vi "Configure.vi"(8 "error in":errorcluster, 10 "name":string, 11 "nPAS in":refnum<class "nPAS.lvclass">) -> (0 "error out":errorcluster, 3 "nPAS out":refnum<class "nPAS.lvclass">)   [LabVIEW 2015, in "nPAS.lvclass"]
doc: "Configure the instrument class. If there is no config file specified, an error"
uses:
  nPAS.lvclass
  Session/Raw FPGA/FPGA Session.lvclass
  Session/Raw FPGA/FPGA Session.lvclass/FPGA Session.ctl
  Reusable/Instrument/Instrument.lvclass/Instrument.ctl
  Reusable/PAS/Main/PAS.lvclass/PAS.ctl
  nPAS.lvclass/nPAS.ctl
  Session/Raw FPGA/Read FPGA Ref.vi
  Reusable/Instrument/Read Cfg Session.vi
  Reusable/PAS/Main/Read Chirp.vi
  Reusable/Instrument/Read Log Session.vi
  Reusable/PAS/Main/Get Speaker State.vi
  <vilib>/Utility/config.llb/Read Key (Double).vi
  <vilib>/Utility/config.llb/Read Key (String).vi
  <vilib>/rvi/interface/common/niFpgaWaitOnOcc.vi
  <vilib>/Utility/error.llb/Error Cluster From Error Code.vi
  <vilib>/rvi/errors/niLvFpgaAdjustHostInterfaceError.vi
  Reusable/PAS/Main/PAS.lvclass
  FPGA Ref.ctl
  <userlib>/_Session Fwk/Session - Root.lvclass
  <vilib>/rvi/interface/nirviMethod/nirviMethod.xnode
  FPGA Bitfiles/NickIO.lvbitx
  <vilib>/rvi/interface/nirviReadWriteControl/nirviReadWriteControl.xnode
  FPGA/PAS Modulation.ctl
  <vilib>/FPGAPlugInAG/cRIO-9081/niLvFpga_ConfigureFifo_cRIO-9081.vi
  <vilib>/rvi/errors/niLvFpgaMergeErrorWithErrorCode.vi
  <vilib>/FPGAPlugInAG/cRIO-9081/niLvFpga_StartFifo_cRIO-9081.vi
  Reusable/Session Log/System Log.lvclass
  Reusable/Session APIs/File Access/Config Data/Config Data.lvclass
  <vilib>/Utility/config.llb/NI_LVConfig.lvlib
  NiFpgaLv.dll
  <vilib>/FPGAPlugInAG/cRIO-9081/niLvFpga_WriteFifo_cRIO-9081.vi
panel:
  out "Actual Depth 2":u32
  out "Actual Depth":u32
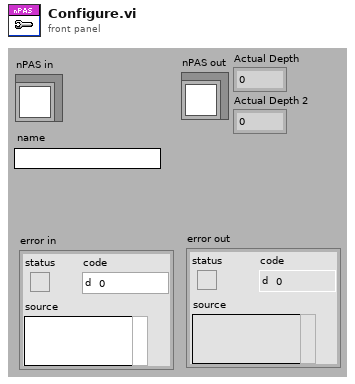
[diagram p1: front panel]
types:
  T1 = cluster{"f0":fxp<+,32,0>, "Mod":enum16{"Sine", "Square"}, "Vscale":fxp<+,32,0>, "Offset":i16}
  T2 = typedef "Session - Root.lvclass/Session Handle.ctl" = refnum<data-value>
  T3 = typedef "FPGA Ref.ctl" = refnum<k20>
  T4 = typedef "NI_LVConfig.lvlib/Config Data RefNum.ctl" = refnum<k1>
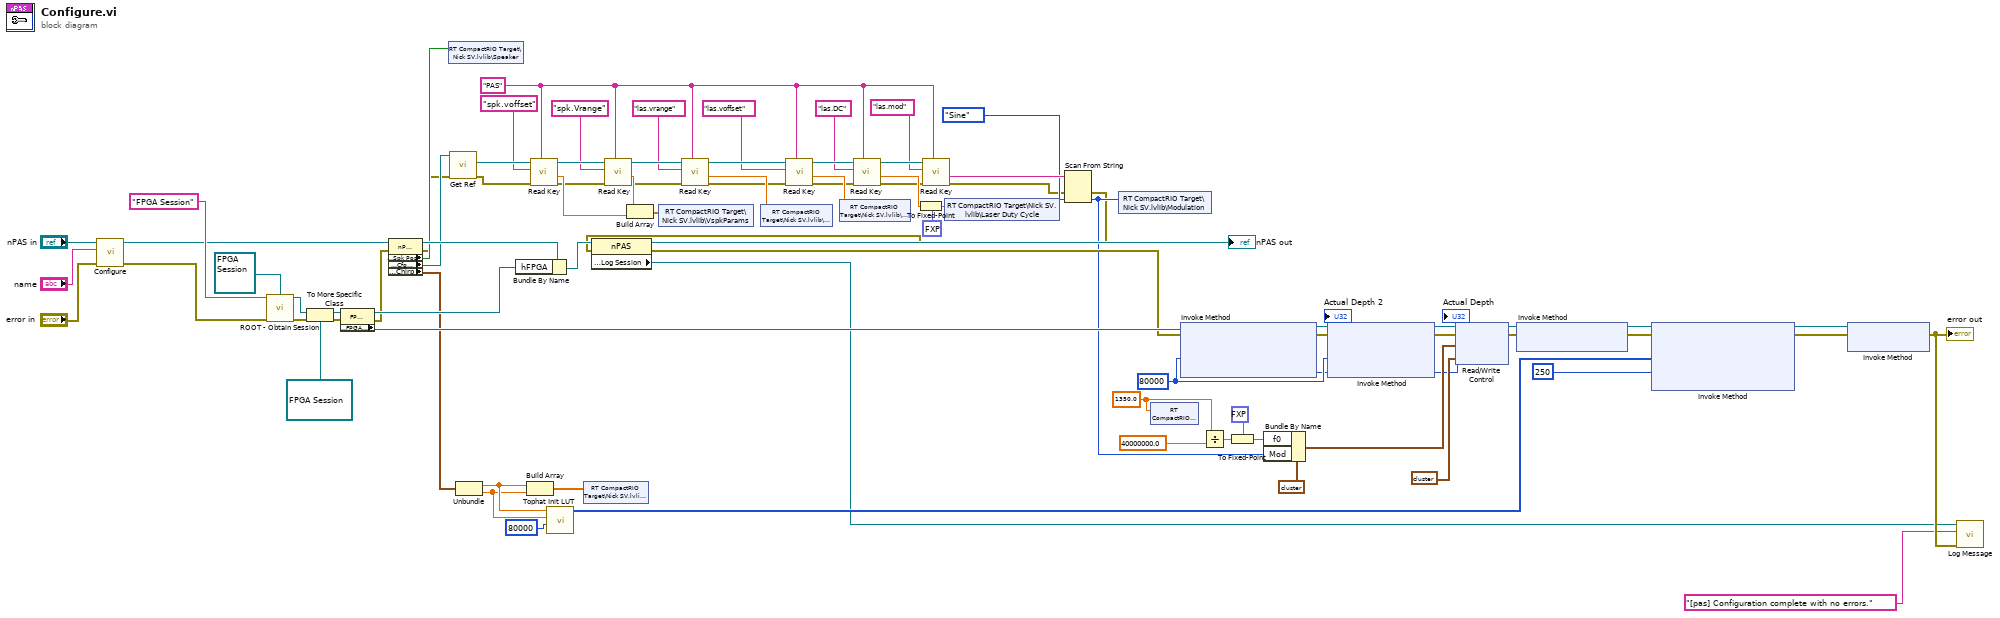
[diagram p0: block diagram]
diagram:
  w28 = "PAS" ("section")
  w59 = 1350.0 ("x")
  w73 = u32 80000 ("Requested Depth")
  n1 = call-parent "Configure.vi"("error in"="error in", "name"="name", "PAS in"="nPAS in") -> ("error out"=w64:errorcluster, "PAS out"=w54:refnum<class "nPAS.lvclass">)  [unwired: 7 in]
  n2 = call <userlib>:"ROOT - Obtain Session.vi"("Session Name ()"="FPGA Session", "OBJ - Session"=refnum<class "FPGA Session.lvclass"> refnum ("FPGA Session.lvclass"), "error in (no error)"=w64) -> ("Session Handle"=w78:T2, "error out"=w77:errorcluster)  [unwired: 10 in, 1 out]
  n3 = To More Specific Class(target class=refnum<data-value> refnum ("hFPGA"), reference=w78, error in=w77) -> (specific class reference=w81:refnum<data-value>, error out=w76:errorcluster)
  n4 = property class="FPGA Session"(reference=w81, error in=w76) -> (reference out=w75:refnum<data-value>, error out=w10:errorcluster, "Accessors:FPGA Ref"=w74:T3)
  n5 = property class="nPAS"(reference=w54, error in=w10) -> (reference out=w53:refnum<class "nPAS.lvclass">, error out=w3:errorcluster, "Data Access:Spk Pos"=w50:bool, "Accessors:Cfg Session"=w49:T2, "Data Access:Chirp"=w9:cluster{"f_center":dbl, "bandwidth":dbl})
  n6 = shared-variable "RT CompactRIO Target\\Nick SV.lvlib\\Speaker"(w50) -> ()  [unwired: 1 in, 1 out]
  n7 = call "Get Ref.vi"("error in"=w3, "Session Handle In"=w49) -> ("error out"=w8:errorcluster, "Ref"=w48:T4)  [unwired: 7 in, 1 out]
  n8 = Unbundle(w9) -> ("f_center"=w52:dbl, "bandwidth"=w51:dbl)
  n9 = Bundle By Name(cluster=w53, "hFPGA"=w75) -> (w62:refnum<class "nPAS.lvclass">)
  n10 = Build Array(w52, w51) -> (w60:dbl[])
  n11 = call-poly <vilib>:"Read Key.vi"("section"=w28, "error in (no error)"=w8, "key"="spk.voffset" ("section"), "refnum"=w48) -> ("error out"=w7:errorcluster, "value"=w44:dbl, "refnum out"=w47:T4)  [unwired: 4 in, 1 out]
  n12 = call "Tophat Init LUT.vi"("Number of  Elements"=80000, "Df"=w51, "f0"=w52) -> ("Init Data Out"=w65:i16[])  [unwired: 6 in]
  n13 = shared-variable "RT CompactRIO Target\\Nick SV.lvlib\\Chirp"(w60) -> ()  [unwired: 1 in, 1 out]
  n14 = call-poly <vilib>:"Read Key.vi"("section"=w28, "error in (no error)"=w7, "key"="spk.Vrange", "refnum"=w47) -> ("error out"=w6:errorcluster, "value"=w43:dbl, "refnum out"=w41:T4)  [unwired: 4 in, 1 out]
  n15 = Build Array(w43, w44) -> (w42:dbl[])
  n16 = shared-variable "RT CompactRIO Target\\Nick SV.lvlib\\VspkParams"(w42) -> ()  [unwired: 1 in, 1 out]
  n17 = call-poly <vilib>:"Read Key.vi"("section"=w28, "error in (no error)"=w6, "key"="las.vrange", "refnum"=w41) -> ("error out"=w5:errorcluster, "value"=w36:dbl, "refnum out"=w40:T4)  [unwired: 4 in, 1 out]
  n18 = shared-variable "RT CompactRIO Target\\Nick SV.lvlib\\Vrange"(w36) -> ()  [unwired: 1 in, 1 out]
  n19 = call-poly <vilib>:"Read Key.vi"("section"=w28, "error in (no error)"=w5, "key"="las.voffset", "refnum"=w40) -> ("error out"=w34:errorcluster, "value"=w37:dbl, "refnum out"=w35:T4)  [unwired: 4 in, 1 out]
  n20 = shared-variable "RT CompactRIO Target\\Nick SV.lvlib\\Voffset"(w37) -> ()  [unwired: 1 in, 1 out]
  n21 = call-poly <vilib>:"Read Key.vi"("section"=w28, "error in (no error)"=w34, "key"="las.DC", "refnum"=w35) -> ("error out"=w27:errorcluster, "value"=w32:dbl, "refnum out"=w29:T4)  [unwired: 4 in, 1 out]
  n22 = To Fixed-Point(fixed-point type=fxp<+,32,0> 0.5 ("Laser Duty Cycle"), number=w32) -> (fixed-point=w30:fxp<+,32,0>)
  n23 = call-poly <vilib>:"Read Key.vi"("section"=w28, "error in (no error)"=w27, "key"="las.mod", "refnum"=w29) -> ("error out"=w22:errorcluster, "value"=w25:string)  [unwired: 4 in, 2 out]
  n24 = shared-variable "RT CompactRIO Target\\Nick SV.lvlib\\Laser Duty Cycle"(w30) -> ()  [unwired: 1 in, 1 out]
  n25 = Scan From String(input string=w25, error in=w22, default 1=enum16{"Sine", "Square"}."Sine" ("Mod")) -> (error out=w2:errorcluster, output 1=w23:enum16{"Sine", "Square"})  [unwired: 2 in, 2 out]
  n26 = property class="nPAS"(reference=w62, error in=w2) -> (reference out=→"nPAS out":refnum<class "nPAS.lvclass">, error out=w57:errorcluster, "Accessors:Log Session"=w56:T2)
  n27 = shared-variable "RT CompactRIO Target\\Nick SV.lvlib\\Modulation"(w23) -> ()  [unwired: 1 in, 1 out]
  n28 = shared-variable "RT CompactRIO Target\\Nick SV.lvlib\\f0"(w59) -> ()  [unwired: 1 in, 1 out]
  n29 = xnode "Invoke Method"("FPGA VI Reference In"=w74, "error in"=w57, "Requested Depth"=w73) -> ("FPGA VI Reference Out"=w21:T3, "error out"=w20:errorcluster, "Actual Depth"=→"Actual Depth 2":u32)
  n30 = Divide(x=w59, y=40000000.0) -> (x/y=w71:dbl)
  n31 = To Fixed-Point(fixed-point type=fxp<+,32,0> 0.0 ("f0"), number=w71) -> (fixed-point=w68:fxp<+,32,0>)
  n32 = Bundle By Name(cluster=T1 {"f0"=0.0, "Mod"=enum."Sine", "Vscale"=0.5, "Offset"=0} ("Wave"), "f0"=w68, "Mod"=w23) -> (w67:T1)
  n33 = xnode "Invoke Method"("FPGA VI Reference In"=w21, "error in"=w20, "Requested Depth"=w73) -> ("FPGA VI Reference Out"=w19:T3, "error out"=w14:errorcluster, "Actual Depth"=→"Actual Depth":u32)
  n34 = xnode "Read/Write Control"("FPGA VI Reference In"=w19, "error in"=w14, "Wave"=w67, "Speaker"=cluster{"Vscale":fxp<+,32,0>, "Offset":i16} {"Vscale"=0.10000000009313226, "Offset"=0}) -> ("FPGA VI Reference Out"=w18:T3, "error out"=w13:errorcluster)
  n35 = xnode "Invoke Method"("FPGA VI Reference In"=w18, "error in"=w13) -> ("FPGA VI Reference Out"=w17:T3, "error out"=w12:errorcluster)
  n36 = xnode "Invoke Method"("FPGA VI Reference In"=w17, "error in"=w12, "Data"=w65, "Timeout (ms)"=250) -> ("FPGA VI Reference Out"=w16:T3, "error out"=w11:errorcluster)  [unwired: 1 out]
  n37 = xnode "Invoke Method"("FPGA VI Reference In"=w16, "error in"=w11) -> ("error out"=w58:errorcluster)  [unwired: 1 out]
  "error out" <- w58
  n38 = call "Log Message.vi"("error in"=w58, "MSG In"="[pas] Configuration complete with no errors.", "session in"=w56) -> ()  [unwired: 7 in, 2 out]
